vi "FlexRay_SignalValue_Conver_Raw.vi"(9 "Signal_Value":dbl, 10 "TFlexRaySignal":T1, 11 "data in":u8[](array[numeric])) -> (3 "data":u8[](array[numeric]))   [LabVIEW 2014]
uses:
  Typedef/FlexRay/TFlexRaySignal.ctl
panel:
  out "Boolean array":bool[](array[boolean])
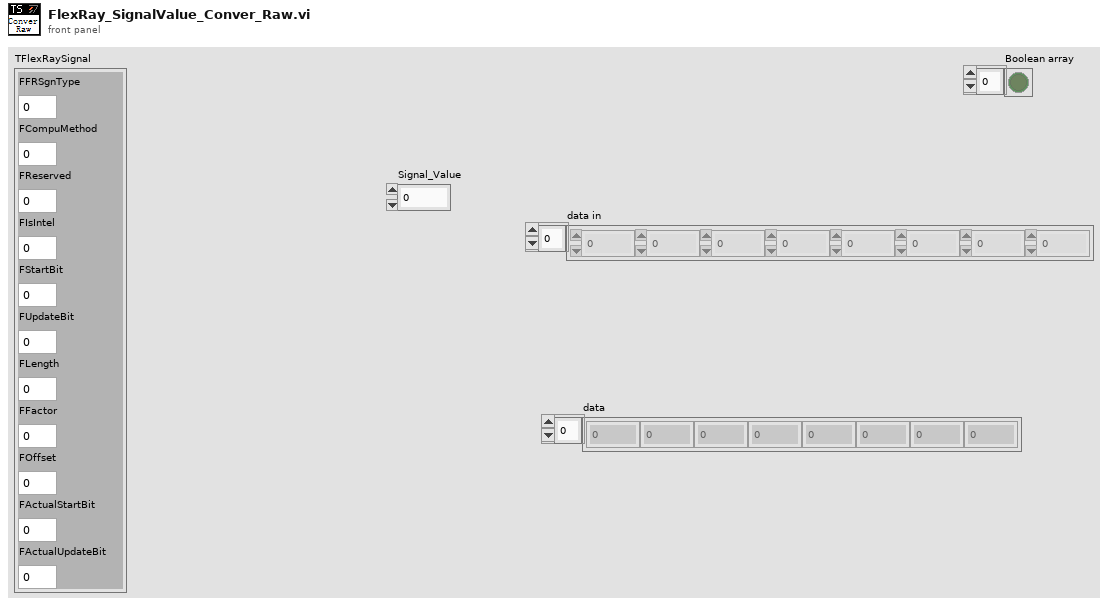
[diagram p1: front panel]
types:
  T1 = typedef "TFlexRaySignal.ctl" = cluster{"FFRSgnType":u8, "FCompuMethod":u8, "FReserved":u8, "FIsIntel":u8, "FStartBit":i32, "FUpdateBit":i32, "FLength":i32, "FFactor":dbl, "FOffset":dbl, "FActualStartBit":i32, "FActualUpdateBit":i32}
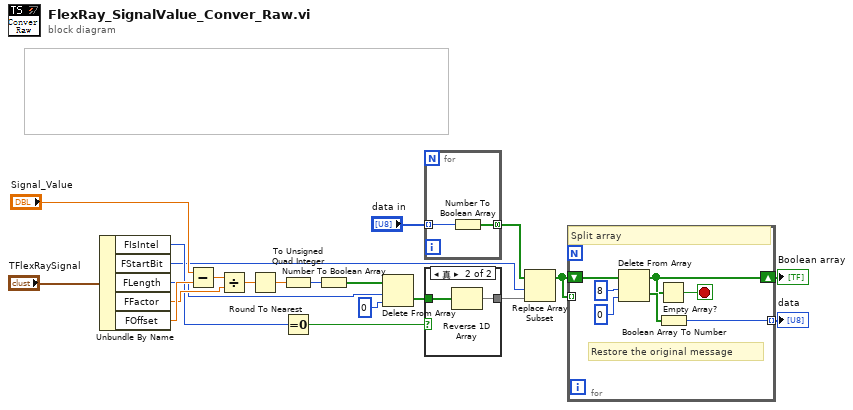
[diagram p0: block diagram]
diagram:
  n1 = Unbundle By Name("TFlexRaySignal") -> ("FIsIntel"=w17:u8, "FStartBit"=w14:i32, "FLength"=w8:i32, "FFactor"=w18:dbl, "FOffset"=w20:dbl)
  n2 = Subtract(x="Signal_Value", y=w20) -> (x-y=w19:dbl)
  n3 = Divide(x=w19, y=w18) -> (x/y=w13:dbl)
  n4 = Round To Nearest(number=w13) -> (nearest integer value=w6:dbl)
  n5 = To Unsigned Quad Integer(1:w6) -> (0:w7:u64)
  n6 = Equal To 0?(x=w17) -> (x = 0?=w16:bool)
  n7 = Number To Boolean Array(number=w7) -> (Boolean array=w12:bool[])
  n8 = Delete From Array(array=w12, length=w8, index=0 ("索引")) -> (deleted portion=w11:bool[])  [unwired: 1 out]
  n9 = for {
    tunnel: "data in" -> [w23] mode=indexing
    tunnel: [w22] -> w15 mode=concatenating
    n10 = Number To Boolean Array(number=w23) -> (Boolean array=w22:bool[])
  }
  n11 = case shown="真" w16 {
    tunnel: w11 -> [w24 w26]
    tunnel: [w24 w25] -> w2
    frame False {
    }
    frame True {
      n12 = Reverse 1D Array(array=w26) -> (reversed array=w25:bool[])
    }
  }
  n13 = Replace Array Subset(array=w15, new element=w2, index=w14) -> (w5:bool[])
  n14 = for {
    tunnel: w5 -> [_] mode=indexing
    shift-right: [w27] -> w4
    shift-left: w5 -> [w29]
    tunnel: [w33] -> w3 mode=indexing
    stop <- w28 stop-if-true
    # "Restore the original message"
    # "Split array"
    n15 = Delete From Array(array=w29, length=8 ("长度"), index=0 ("索引")) -> (deleted portion=w31:bool[], array with subset deleted=w27:bool[])
    n16 = Empty Array?(array=w27) -> (empty?=w28:bool)
    n17 = Boolean Array To Number(Boolean array=w31) -> (number=w33:u32)
  }
  "data" <- w3
  "Boolean array" <- w4
